vi "Init.vi"(10 "Actor":refnum<class "Actor.lvclass">) -> (3 "Last Ack Msg out":refnum<class "Last Ack Msg.lvclass">)   [LabVIEW 2020, in "jettl.lvlib" / "Last Ack Msg.lvlib" / "Last Ack Msg.lvclass"]
uses:
  Last Ack Msg.lvclass
  Actor/Actor/Actor.lvclass
  Last Ack Msg.lvclass/Last Ack Msg.ctl
  Sender/Sender/Sender.lvclass
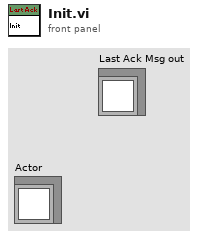
[diagram p1: front panel]
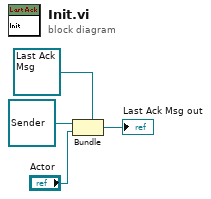
[diagram p0: block diagram]
diagram:
  n1 = Bundle "Bundle"(cluster=refnum<class "Last Ack Msg.lvclass"> refnum ("Last Ack Creator Queue Msg Strategy out"), refnum<class "Sender.lvclass"> refnum ("Sender"), "Actor") -> (→"Last Ack Msg out":refnum<class "Last Ack Msg.lvclass">)
